vi "SetWaveformUnit.vi"(8 "error in (no error)":errorcluster, 10 "Unit":string, 11 "Waveform in":waveform(sgl)) -> (0 "error out":errorcluster, 3 "Waveform out":waveform(sgl))   [LabVIEW 2017]
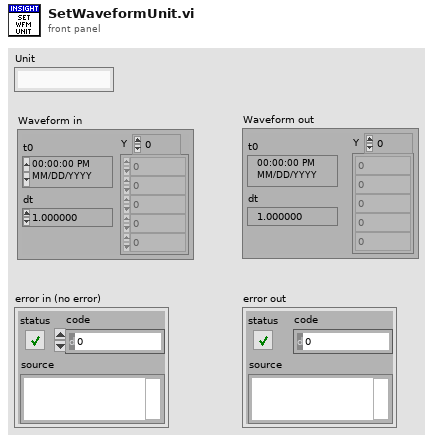
[diagram p1: front panel]
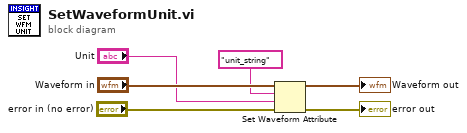
[diagram p0: block diagram]
diagram:
  n1 = Set Waveform Attribute(4:"error in (no error)", 5:"Unit", 6:"unit_string" ("name"), 7:"Waveform in") -> (0:→"error out":errorcluster, 3:→"Waveform out":waveform(sgl))  [unwired: 1 out]
